vi "Set State.vi"(8 "error in (no error)":errorcluster, 10 "State":T1, 11 "Incoming in":refnum<class "Incoming.lvclass">) -> (0 "error out":errorcluster, 3 "Incoming out":refnum<class "Incoming.lvclass">)   [LabVIEW 2022 SP3, in "Incoming.lvlib" / "Incoming.lvclass"]
uses:
  Incoming.lvclass
  Elevator Controller/Elevator Controller/States -Enum.ctl
  Elevator Controller/Elevator Controller/Elevator Controller.lvclass
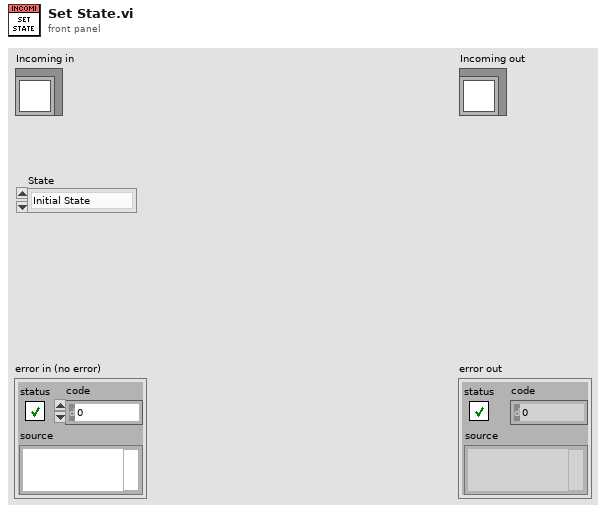
[diagram p1: front panel]
types:
  T1 = typedef "Elevator Controller.lvlib/Elevator Controller.lvclass/States -Enum.ctl" = enum16{"Initial State", "Wait for First Request", "Start and Move State", "Analysis State", "Continue Travel State", "Stop at Floor", "Open and Close Door Sequence", "No Request Remaining", "Emergency Call", "Terminate Process", ""}
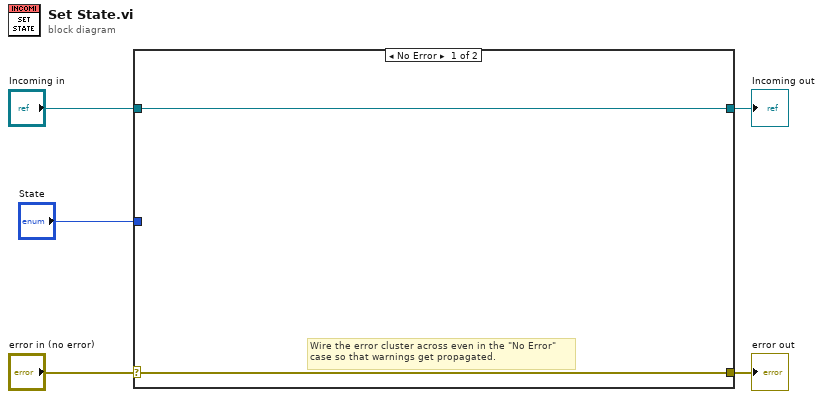
[diagram p0: block diagram]
diagram:
  n1 = case shown="No Error" "error in (no error)" {
    selector: "error in (no error)" -> [w6 w9]
    tunnel: [w6 w9] -> w4
    tunnel: [w7 w8] -> w2
    tunnel: "Incoming in" -> [w7 w8]
    tunnel: "State" -> [_ _]
    frame No Error {
      # "Wire the error cluster across even in the \"No Error\"\ncase so that warnings get propagated."
    }
    frame Error {
    }
  }
  "error out" <- w4
  "Incoming out" <- w2
